vi "Main.vi"(8 "error in":errorcluster, 11 "Second Level Worker in":refnum<class "Second Level Worker.lvclass">) -> (0 "error out":errorcluster, 3 "Second Level Worker out":refnum<class "Second Level Worker.lvclass">)   [LabVIEW 2017, in "Method 1.lvlib" / "Second Level Worker.lvclass"]
doc: "The <b>Queued Message Handler</b> of the Worker that owns this VI."
uses:
  Second Level Worker.lvclass
  C:/Program Files (x86)/National Instruments/LabVIEW 2017/vi.lib/addons/_Workers/Library/Classes/Worker/Worker.lvclass
  Initialization Data.ctl
  Response Cases.ctl
  <vilib>/addons/_Workers/Library/Case Label.ctl
  Second Level Worker.lvclass/Second Level Worker.ctl
  rql_Send Error to Caller.ctl
  <vilib>/addons/_Workers/Library/Classes/Message Queue/Message Queue.lvclass
  <vilib>/addons/_Workers/Library/Workers.lvlib
panel:
  in  "Send Error to Caller":bool
  in  "User Error":errorcluster={"status"=TRUE, "code"=12345, "source"="Hello World! This is an error message."}
  # "Method 1 : Using Public API Responses"
  # "Second Level Worker (Main VI)"
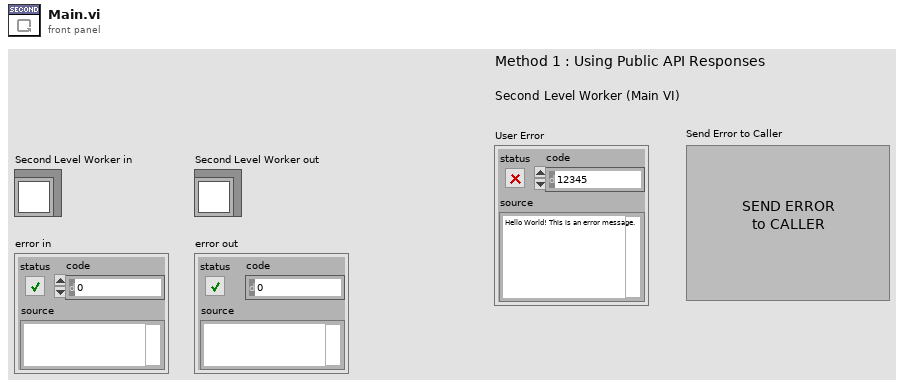
[diagram p1: front panel]
types:
  T1 = typedef "Method 1.lvlib/Second Level Worker.lvclass/Initialization Data.ctl" = cluster{"Response Cases":T2}
  T2 = typedef "Method 1.lvlib/Second Level Worker.lvclass/Response Cases.ctl" = cluster{"subWorker Error":T3}
  T3 = typedef "Workers.lvlib/Case Label.ctl" = string
  T4 = typedef "Method 1.lvlib/Second Level Worker.lvclass/rql_Send Error to Caller.ctl" = cluster{"String":string}
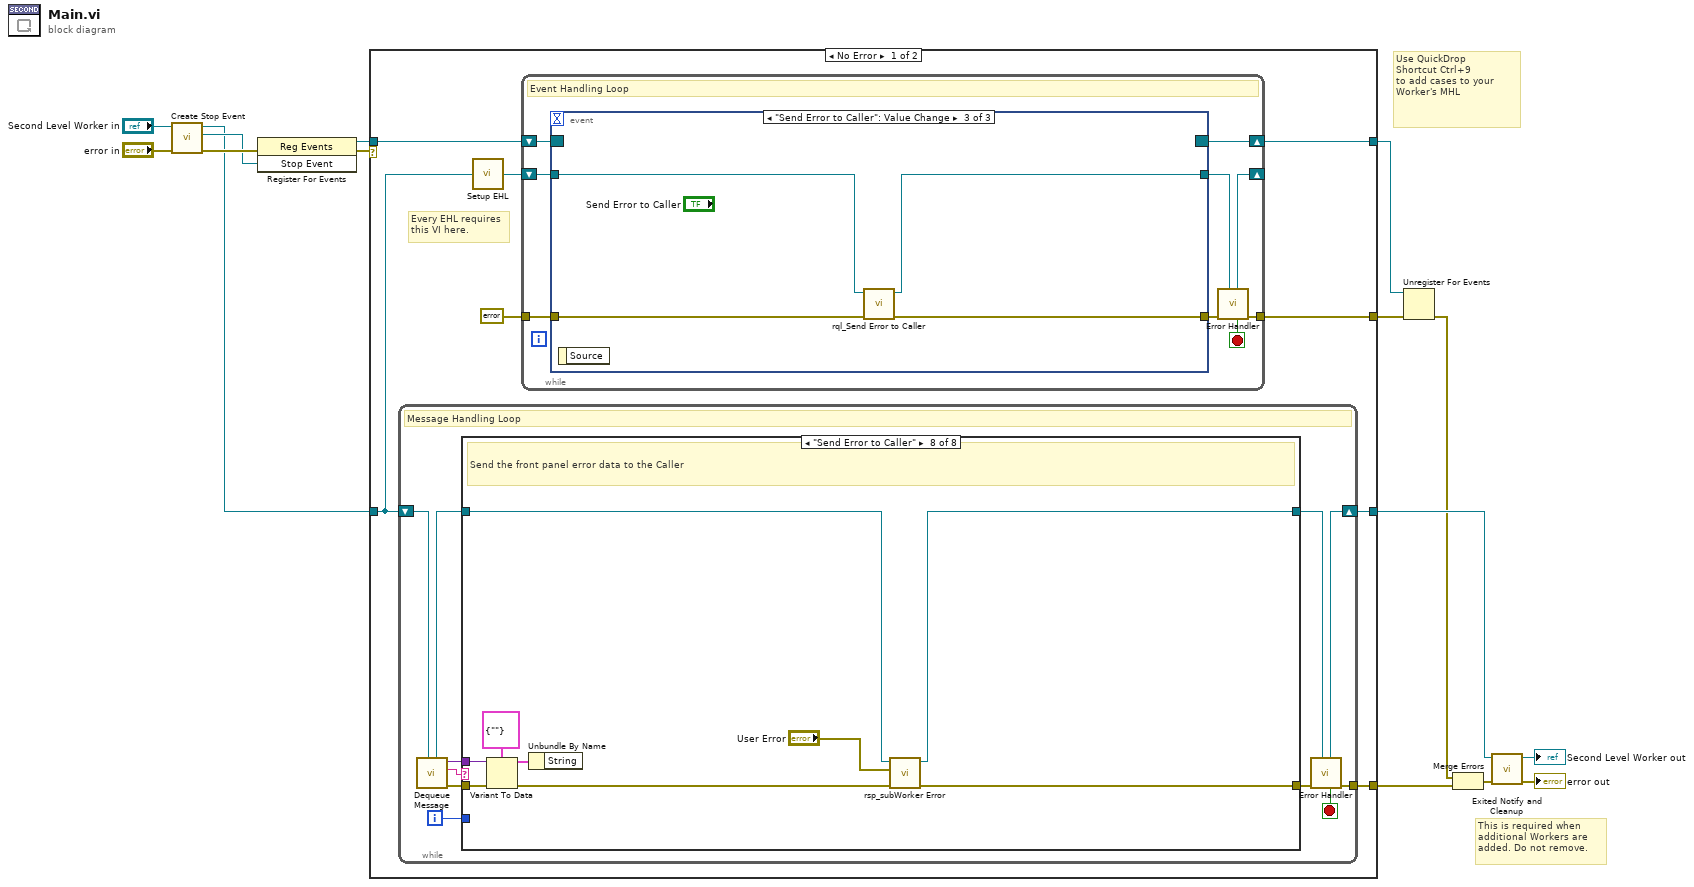
[diagram p0: block diagram]
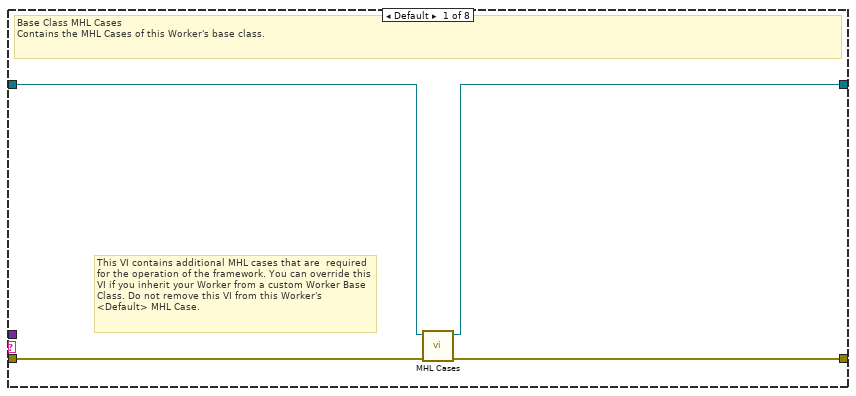
[diagram p2: hidden frame]
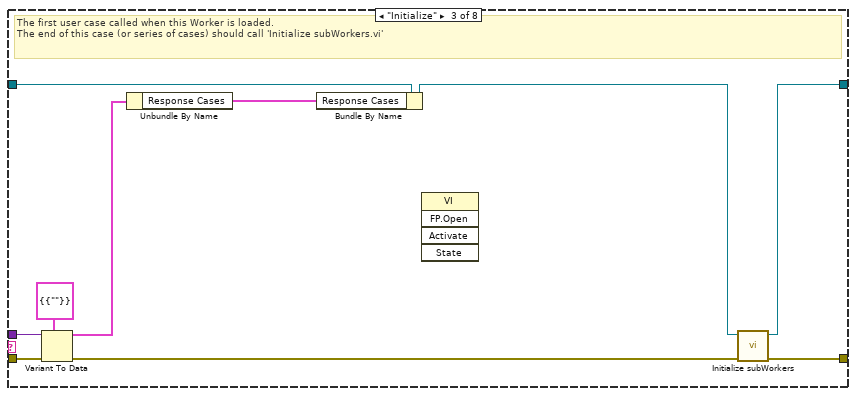
[diagram p4: hidden frame]
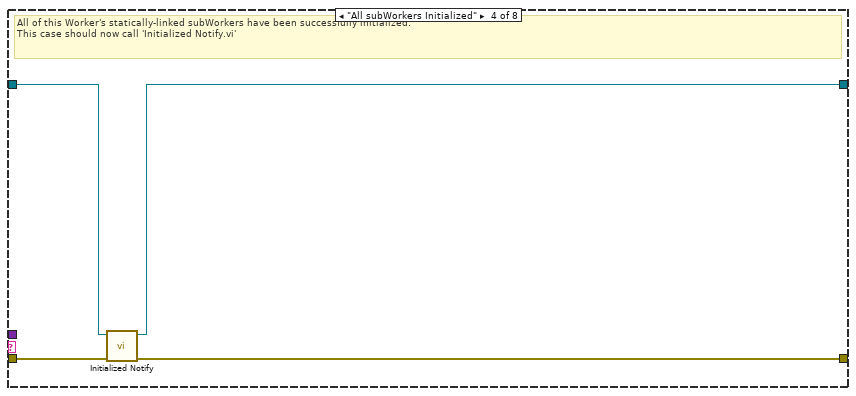
[diagram p5: hidden frame]
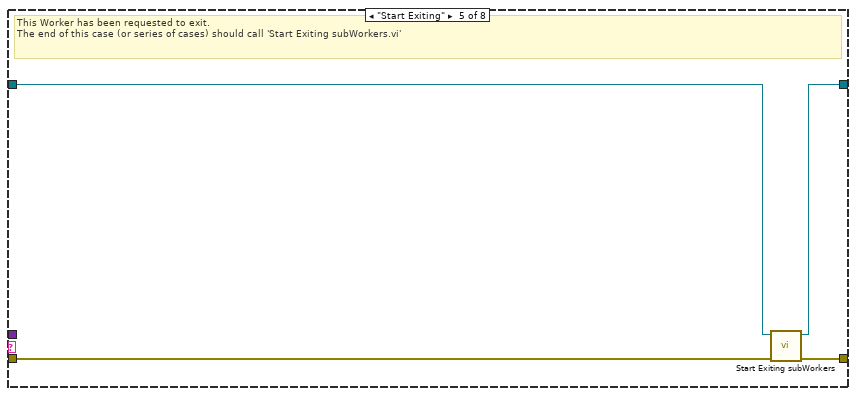
[diagram p6: hidden frame]
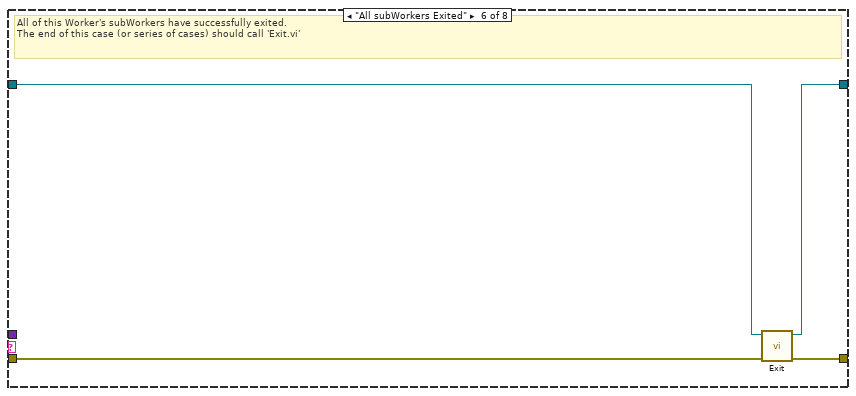
[diagram p7: hidden frame]
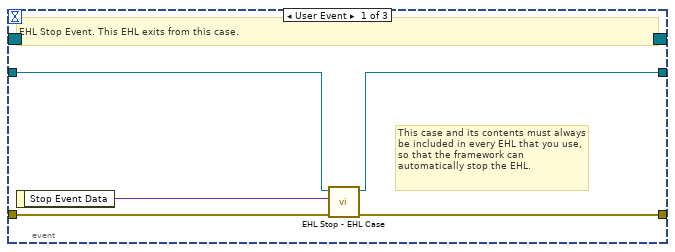
[diagram p9: hidden frame]
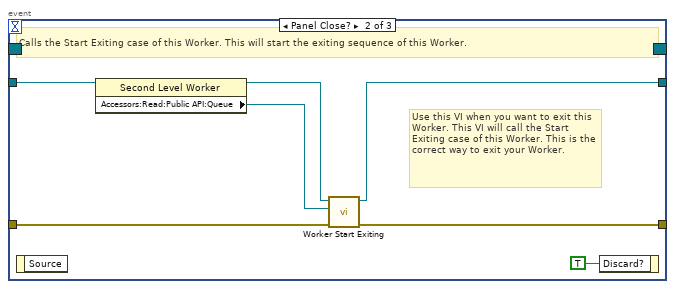
[diagram p10: hidden frame]
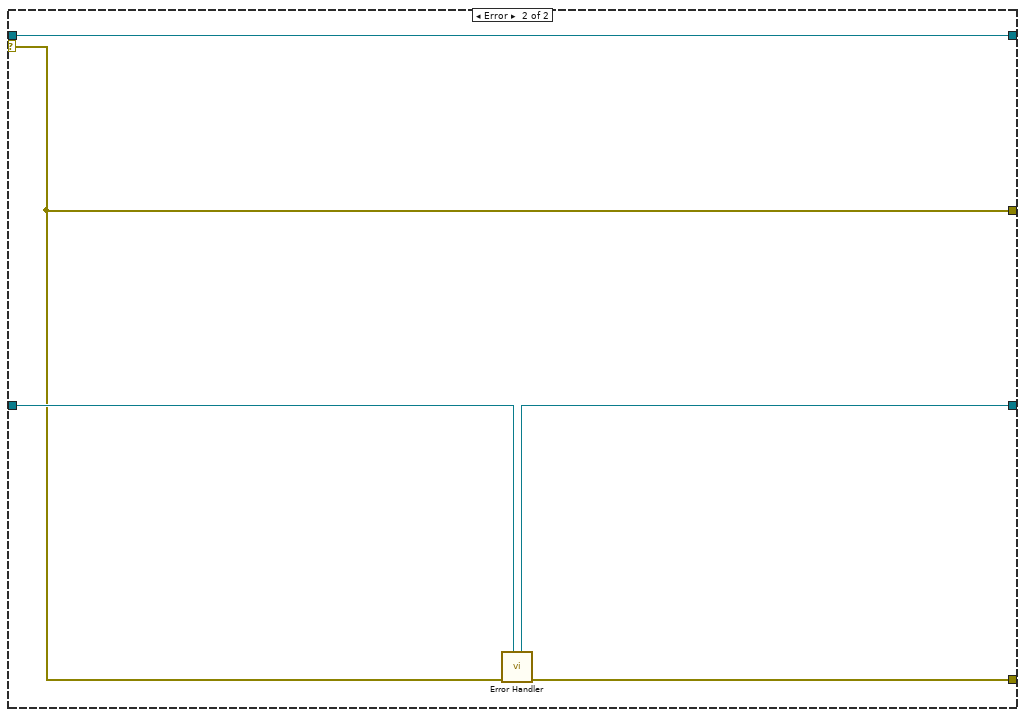
[diagram p11: hidden frame]
diagram:
  # "Use QuickDrop\nShortcut Ctrl+9\nto add cases to your\nWorker's MHL"
  # "This is required when additional Workers are added. Do not remove."
  n1 = call-dynamic "Create Stop Event.vi"("error in"="error in", "Worker"="Second Level Worker in") -> ("error out"=w5:errorcluster, "Stop Event"=w4:refnum<user-event>, "Worker out"=w3:refnum<class "Second Level Worker.lvclass">)  [unwired: 7 in]
  n2 = register-events(error in=w5, w4) -> (reference out=w10:refnum<event-registration>, error out=w7:errorcluster)  [unwired: 1 in]
  n3 = case shown="No Error" w7 {
    tunnel: w3 -> [w19 w102]
    tunnel: [w23 w103] -> w14
    tunnel: [w22 w101] -> w15
    selector: w7 -> [_ w99]
    tunnel: w10 -> [w18 w100]
    tunnel: [w17 w99] -> w9
    tunnel: [w16 w100] -> w8
    frame No Error {
      # "Every EHL requires\nthis VI here."
      n4 = while {
        shift-right: [w32] -> w22
        shift-left: w19 -> [w34]
        tunnel: [w33] -> w23
        i -> [w25]
        stop <- w26 stop-if-true
        # "Message Handling Loop"
        n5 = call-dynamic "Dequeue Message.vi"("Worker"=w34) -> ("error out"=w31:errorcluster, "Case out"=w27:string, "Data out"=w24:variant, "Worker out"=w29:refnum<class "Second Level Worker.lvclass">)  [unwired: 6 in, 1 out]
        n6 = case "Worker MHL Case Structure (DO NOT CHANGE LABEL NAME)" shown="\"Send Error to Caller\"" w27 {
          tunnel: w31 -> [w38 w39 w48 w54 w55 w62 w64 w73]
          tunnel: [w37 w39 w50 w53 w58 w61 w64 w69] -> w30
          tunnel: w29 -> [w36 w40 w47 w52 w56 w60 w63 w68]
          tunnel: [w35 w40 w49 w51 w57 w59 w63 w67] -> w28
          tunnel: w25 -> [_ _ _ _ _ _ _ _]
          tunnel: w24 -> [_ _ w45 _ _ _ _ w71]
          frame Default {
            # "This VI contains additional MHL cases that are  required for the operation of the framework. You can override this VI if you inherit your Worker from a custom Worker Base Class. Do not remove this VI from this Worker's <Default> MHL Case."
            # "Base Class MHL Cases\nContains the MHL Cases of this Worker's base class."
            n7 = call-dynamic "MHL Cases.vi"("error in"=w38, "Worker in"=w36) -> ("error out"=w37:errorcluster, "Worker out"=w35:refnum<class "Second Level Worker.lvclass">)  [unwired: 8 in]
          }
          frame "------------ FRAMEWORK CASES -----------" {
            # "Start of Workers Framework Cases"
          }
          frame "Initialize" {
            # "The first user case called when this Worker is loaded.\nThe end of this case (or series of cases) should call 'Initialize subWorkers.vi'"
            n8 = Variant To Data(error in=w48, type=T1 {"Response Cases"={"subWorker Error"=""}} ("Cluster"), Variant=w45) -> (data=w43:T1, error out=w46:errorcluster)
            n9 = Unbundle By Name(w43) -> ("Response Cases"=w42:T2)
            n10 = Bundle By Name(cluster=w47, "Response Cases"=w42) -> (w44:refnum<class "Second Level Worker.lvclass">)
            n11 = invoke class="VI" method="FP.Open"() -> ()  [unwired: 5 in, 5 out]
            n12 = call-dynamic "Initialize subWorkers.vi"("error in"=w46, "Worker"=w44) -> ("error out"=w50:errorcluster, "dup Worker out"=w49:refnum<class "Second Level Worker.lvclass">)  [unwired: 8 in]
          }
          frame "All subWorkers Initialized" {
            # "All of this Worker's statically-linked subWorkers have been successfully initialized.\nThis case should now call 'Initialized Notify.vi'"
            n13 = call-dynamic "Initialized Notify.vi"("error in"=w54, "Worker"=w52) -> ("error out"=w53:errorcluster, "dup Worker out"=w51:refnum<class "Second Level Worker.lvclass">)  [unwired: 8 in]
          }
          frame "Start Exiting" {
            # "This Worker has been requested to exit. \nThe end of this case (or series of cases) should call 'Start Exiting subWorkers.vi'"
            n14 = call-dynamic "Start Exiting subWorkers.vi"("error_in"=w55, "Worker"=w56) -> ("error out"=w58:errorcluster, "dup Worker out"=w57:refnum<class "Second Level Worker.lvclass">)  [unwired: 8 in]
          }
          frame "All subWorkers Exited" {
            # "All of this Worker's subWorkers have successfully exited. \nThe end of this case (or series of cases) should call 'Exit.vi'"
            n15 = call-dynamic "Exit.vi"("error_in"=w62, "Worker"=w60) -> ("error out"=w61:errorcluster, "dup Worker out"=w59:refnum<class "Second Level Worker.lvclass">)  [unwired: 8 in]
          }
          frame "------------- LOCAL API CASES -------------" {
            # "Start of Workers Local API Cases"
          }
          frame "Send Error to Caller" {
            # "Send the front panel error data to the Caller"
            n16 = Variant To Data(error in=w73, type=T4 {"String"=""} ("Data"), Variant=w71) -> (data=w70:T4, error out=w66:errorcluster)
            n17 = Unbundle By Name(w70) -> ()  [unwired: 1 out]
            n18 = call "rsp_subWorker Error.vi"("error in"=w66, "Data in"="User Error", "Second Level Worker in"=w68) -> ("error out"=w69:errorcluster, "dup Second Level Worker out"=w67:refnum<class "Second Level Worker.lvclass">)  [unwired: 7 in]
          }
        }
        n19 = call-dynamic "Error Handler.vi"("Worker"=w28, "error_in"=w30) -> ("error out"=w33:errorcluster, "Stop Loop"=w26:bool, "Worker out"=w32:refnum<class "Second Level Worker.lvclass">)  [unwired: 7 in]
      }
      n20 = call-dynamic "Setup EHL.vi"("Worker"=w19) -> ("Worker out"=w20:refnum<class "Second Level Worker.lvclass">)  [unwired: 14 in]
      n21 = while "Event Handling Loop" {
        shift-right: [w82] -> w16
        shift-left: w18 -> [w81]
        tunnel: [w77] -> w17
        tunnel: errorcluster {"status"=FALSE, "code"=0, "source"=""} ("error constant") -> [w79]
        shift-right: [w75] -> _
        shift-left: w20 -> [w80]
        stop <- w74 stop-if-true
        # "Event Handling Loop"
        n22 = event shown="[2] \"Send Error to Caller\": Value Change" {
          selector: w81 -> [_ _ _]
          dyn-events: [_ _ _] -> w82
          timeout: _ -> [_ _ _]
          tunnel: [w86 w93 w97] -> w78
          tunnel: w79 -> [w87 w92 w98]
          tunnel: w80 -> [w85 w91 w96]
          tunnel: [w84 w90 w95] -> w76
          event User Event {
            # "This case and its contents must always be included in every EHL that you use, so that the framework can automatically stop the EHL."
            # "EHL Stop Event. This EHL exits from this case."
            n23 = event-data() -> ("Stop Event Data"=w83:variant)  [unwired: 1 in]
            n24 = call-dynamic "EHL Stop - EHL Case.vi"("error in"=w87, "Stop Event Data"=w83, "Worker"=w85) -> ("error out"=w86:errorcluster, "Worker out"=w84:refnum<class "Second Level Worker.lvclass">)  [unwired: 7 in]
          }
          event Panel Close? {
            # "Use this VI when you want to exit this Worker. This VI will call the Start Exiting case of this Worker. This is the correct way to exit your Worker."
            # "Calls the Start Exiting case of this Worker. This will start the exiting sequence of this Worker."
            n25 = event-data() -> ()  [unwired: 1 in, 1 out]
            n26 = property class="Second Level Worker"(reference=w91) -> (reference out=w89:refnum<class "Second Level Worker.lvclass">, "Accessors:Read:Public API:Queue"=w88:refnum<class "Message Queue.lvclass">)  [unwired: 1 in, 1 out]
            n27 = call-dynamic "Worker Start Exiting.vi"("error_in"=w92, "Message Queue"=w88, "Worker"=w89) -> ("error out"=w93:errorcluster, "dup Worker out"=w90:refnum<class "Second Level Worker.lvclass">)  [unwired: 7 in]
            n28 = event-data ("Event Filter Node")("Discard?"=TRUE) -> ()  [unwired: 1 in, 1 out]
          }
          event "Send Error to Caller": Value Change {
            n29 = event-data() -> ()  [unwired: 1 in, 1 out]
            n30 = call "rql_Send Error to Caller.vi"("error in"=w98, "Second Level Worker in"=w96) -> ("error out"=w97:errorcluster, "dup Second Level Worker out"=w95:refnum<class "Second Level Worker.lvclass">)  [unwired: 8 in]
          }
        }
        n31 = call-dynamic "Error Handler.vi"("Worker"=w76, "error_in"=w78) -> ("error out"=w77:errorcluster, "Stop Loop"=w74:bool, "Worker out"=w75:refnum<class "Second Level Worker.lvclass">)  [unwired: 7 in]
      }
    }
    frame Error {
      n32 = call-dynamic "Error Handler.vi"("Worker"=w102, "error_in"=w99) -> ("error out"=w103:errorcluster, "Worker out"=w101:refnum<class "Second Level Worker.lvclass">)  [unwired: 7 in, 1 out]
    }
  }
  n33 = Unregister For Events(event registration refnum=w8, error in=w9) -> (error out=w6:errorcluster)
  n34 = Merge Errors(w6, w14) -> (w11:errorcluster)
  n35 = call-dynamic "Exited Notify and Cleanup.vi"("error_in"=w11, "Worker"=w15) -> ("error out"=→"error out":errorcluster, "dup Worker out"=→"Second Level Worker out":refnum<class "Second Level Worker.lvclass">)  [unwired: 8 in]
